vi "FindCircle.vi"(5 "Y":dbl format="%#_13g", 7 "X":dbl format="%#_13g", 8 "error in (no error)":errorcluster, 11 "Image 2":T1(plugin-control)) -> (0 "error out":errorcluster, 2 "Circle Descriptor":T2(array[cluster]), 3 "Image Out":T1)   [LabVIEW 2016]
uses:
  <vilib>/vision/Image Controls.llb/IMAQ Image.ctl
  <vilib>/userdefined/High Color/IMAQdx.ctl
  <vilib>/vision/NI_Vision_Development_Module.lvlib
  <vilib>/vision/driver/NI_Vision_Acquisition_Software.lvlib
panel:
  out "Circle Descriptor 2":T2(array[cluster])
  in  "Color Plane":i32(ring)=1 items=["Red", "Green", "Blue", "Hue", "Saturation", "Luminance", "Value", "Intensity"]
  out "Image":T1(plugin-control)
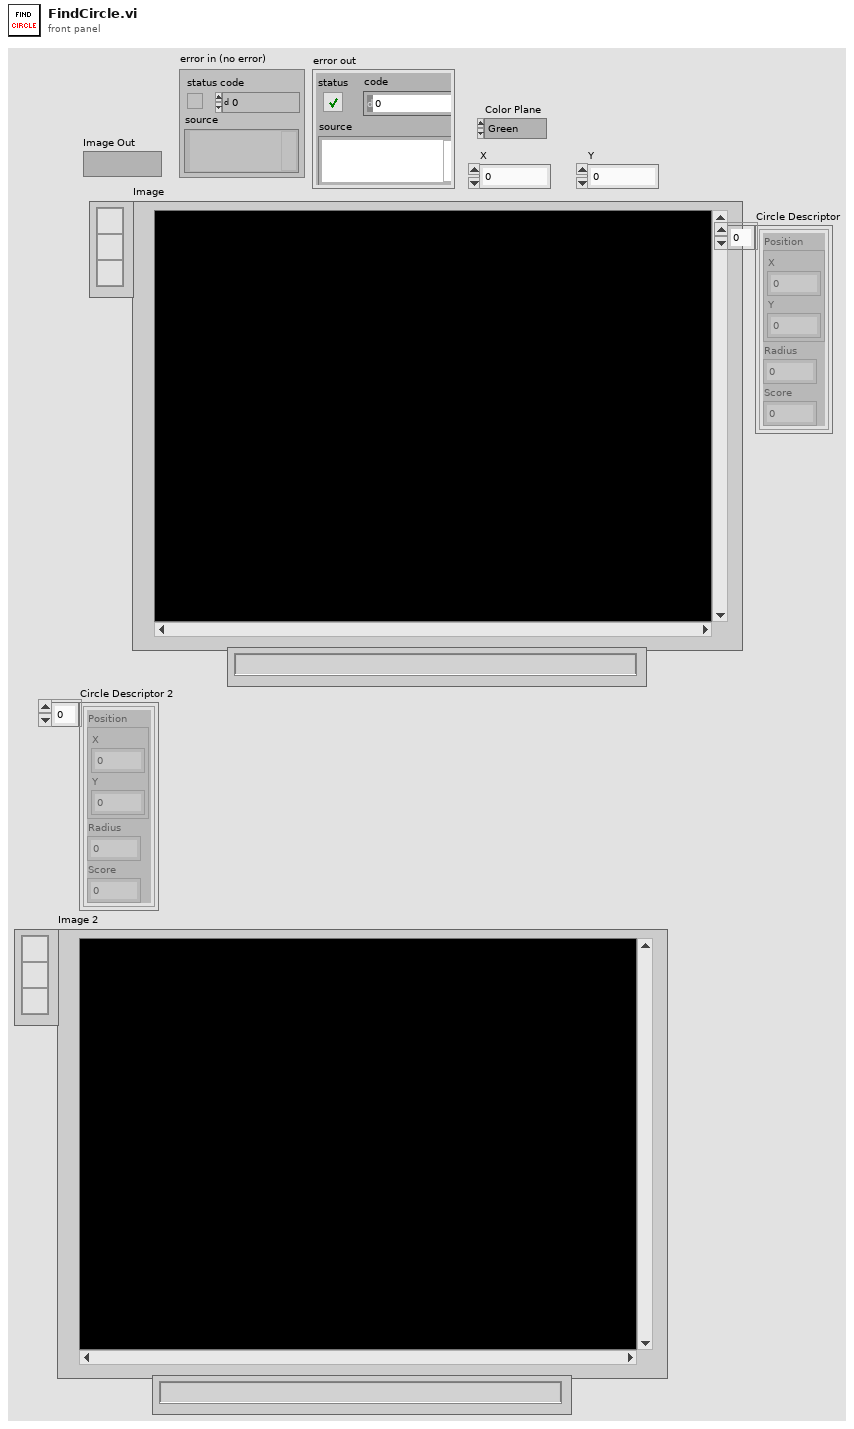
[diagram p1: front panel]
types:
  T1 = typedef "IMAQ Image.ctl" = refnum<image>
  T2 = cluster{"Position":cluster{"X":sgl, "Y":sgl}, "Radius":dbl, "Score":dbl}[]
  T3 = typedef "IMAQdx.ctl" = refnum<k21>
  T4 = typedef "IMAQ Circle" = cluster{"Center X":i32, "Center Y":i32, "Inner Radius":i32, "Outer Radius":i32, "Start Angle":dbl, "End Angle":dbl}
  T5 = typedef "ROI Descriptor" = cluster{"Global Rectangle":i32[], "Contours":cluster{"ID":enum32{"External", "Internal"}, "Type":u32, "Coordinates":i32[]}[]}
  T6 = cluster{"Position":cluster{"X":sgl, "Y":sgl}, "Radius":dbl, "Score":dbl}
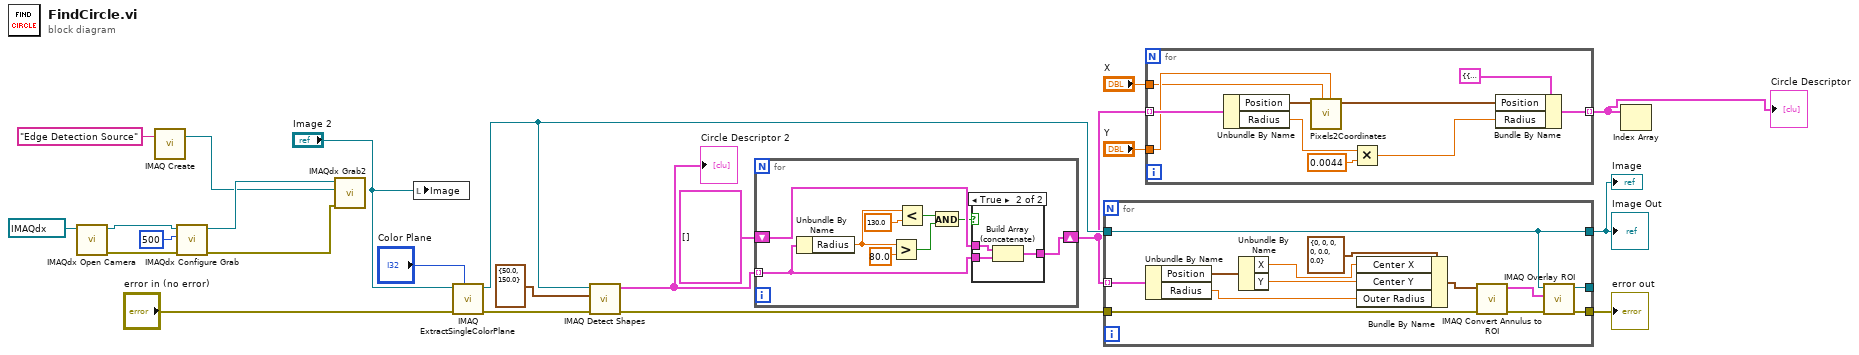
[diagram p0: block diagram]
diagram:
  n1 = call <vilib>:"IMAQdx Open Camera.vi"("Session In"=T3 "cam0") -> ("error out"=w9:errorcluster, "Session Out"=w8:T3)  [unwired: 9 in]
  n2 = call "IMAQ Create"("Image Name"="Edge Detection Source") -> ("New Image"=w3:T1)  [unwired: 4 in, 1 out]
  n3 = call <vilib>:"IMAQdx Configure Grab.vi"("error in"=w9, "Number of Buffers"=u32 500, "Session In"=w8) -> ("error out"=w5:errorcluster, "Session Out"=w6:T3)  [unwired: 7 in]
  n4 = call <vilib>:"IMAQdx Grab2.vi"("error in"=w5, "Image In"=w3, "Session In"=w6) -> ()  [unwired: 5 in, 4 out]
  n5 = local write "Image"("Image 2") -> ()
  n6 = call "IMAQ ExtractSingleColorPlane"("Color Plane"="Color Plane", "error in (no error)"="error in (no error)", "Image Src"="Image 2") -> ("error out"=w22:errorcluster, "Image Dst Out"=w19:T1)  [unwired: 7 in]
  n7 = call-poly "IMAQ Detect Shapes"("error in (no error)"=w22, "Circle Descriptor"=cluster{"Min Radius":dbl, "Max Radius":dbl} {"Min Radius"=50.0, "Max Radius"=150.0}, "Image"=w19) -> ("error out"=w20:errorcluster, "Circles"=w12:T2)  [unwired: 6 in, 1 out]
  "Circle Descriptor 2" <- w12
  n8 = for {
    tunnel: w12 -> [w32] mode=indexing
    shift-right: [w29] -> w16
    shift-left: T2 [] ("Circle Descriptor") -> [w30]
    n9 = Unbundle By Name(w32) -> ("Radius"=w28:dbl)
    n10 = Greater?(x=w28, y=80.0) -> (0:w25:bool)
    n11 = Less?(x=w28, y=130.0) -> (x < y?=w26:bool)
    n12 = And(x=w26, y=w25) -> (x .and. y?=w24:bool)
    n13 = case shown="True" w24 {
      tunnel: w32 -> [_ w35]
      tunnel: w30 -> [w33 w36]
      tunnel: [w33 w34] -> w29
      frame False {
      }
      frame True {
        n14 = Build Array (concatenate)(w36, w35) -> (w34:T2)
      }
    }
  }
  n15 = for {
    tunnel: w16 -> [w49] mode=indexing
    tunnel: w19 -> [w39]
    tunnel: w20 -> [w41]
    tunnel: [w39] -> w13
    tunnel: [w38] -> w17
    tunnel: [w37] -> _
    n16 = Unbundle By Name(w49) -> ("Position"=w48:cluster{"X":sgl, "Y":sgl}, "Radius"=w43:dbl)
    n17 = Unbundle By Name(w48) -> ("X"=w45:sgl, "Y"=w44:sgl)
    n18 = Bundle By Name(cluster=T4 {"Center X"=0, "Center Y"=0, "Inner Radius"=0, "Outer Radius"=0, "Start Angle"=0.0, "End Angle"=0.0} ("Annulus"), "Center X"=w45, "Center Y"=w44, "Outer Radius"=w43) -> (w46:T4)
    n19 = call "IMAQ Convert Annulus to ROI"("error in (no error)"=w41, "Annulus"=w46) -> ("error out"=w40:errorcluster, "ROI Descriptor"=w42:T5)  [unwired: 7 in]
    n20 = call "IMAQ Overlay ROI"("error in (no error)"=w40, "ROI Descriptor"=w42, "Image"=w39) -> ("error out"=w38:errorcluster, "Image Out"=w37:T1)  [unwired: 7 in]
  }
  "Image" <- w13
  "Image Out" <- w13
  "error out" <- w17
  n21 = for {
    tunnel: w16 -> [w59] mode=indexing
    tunnel: [w52] -> w2 mode=indexing
    tunnel: "X" -> [w50]
    tunnel: "Y" -> [w51]
    n22 = Unbundle By Name(w59) -> ("Position"=w54:cluster{"X":sgl, "Y":sgl}, "Radius"=w56:dbl)
    n23 = call "Pixels2Coordinates.vi"("Y"=w51, "X"=w50, "Location (Pixel)"=w54) -> ("output cluster"=w53:cluster{"X":sgl, "Y":sgl})  [unwired: 8 in]
    n24 = Multiply(x=w56, y=0.0044) -> (x*y=w57:dbl)
    n25 = Bundle By Name(cluster=T6 {"Position"={"X"=0.0, "Y"=0.0}, "Radius"=0.0, "Score"=0.0} ("Circle Descriptor"), "Position"=w53, "Radius"=w57) -> (w52:T6)
  }
  "Circle Descriptor" <- w2
  n26 = Index Array(array=w2) -> ()  [unwired: 1 in, 1 out]
